vi "pattern.vi"() -> ()   [LabVIEW 2025]
uses:
  ready/Type Def/steps--ring.ctl
panel:
  out "error out":errorcluster
  in  "error in (no error)":errorcluster
  out "VISA resource name out":refnum<visa-resource-name>
  in  "VISA resource name":refnum<visa-resource-name>
  out "ARC value":string
  out "Resulting command":string
  in  "Step":T1=1 min=1 max=99 step=1
  # "Configure ARC Limit"
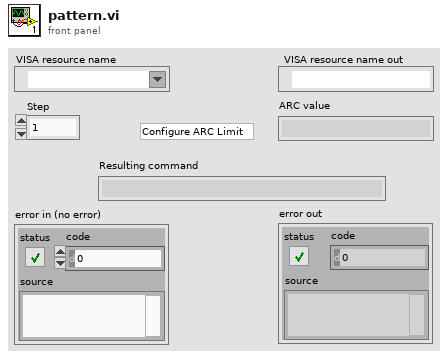
[diagram p1: front panel]
types:
  T1 = typedef "steps--ring.ctl" = u8
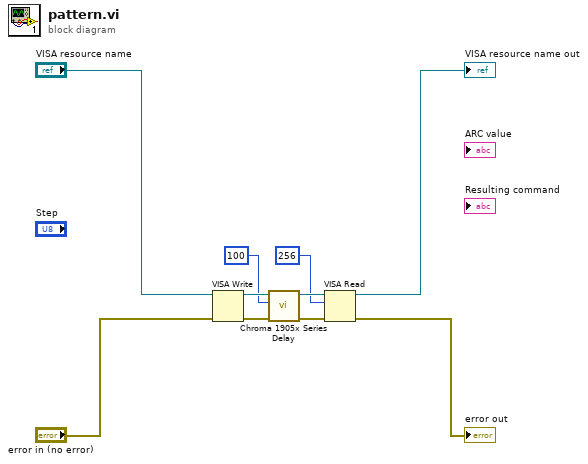
[diagram p0: block diagram]
diagram:
  n1 = VISA Write(VISA resource name="VISA resource name", error in (no error)="error in (no error)") -> (VISA resource name out=w8:refnum<visa-resource-name>, error out=w10:errorcluster)  [unwired: 1 in, 1 out]
  n2 = call "Chroma 1905x Series Delay.vi"("error in (no error)"=w10, "Time Delay [ms]"=u32 100 ("Time Delay ms"), "VISA resource name"=w8) -> ("error out"=w9:errorcluster, "VISA resource name 2"=w7:refnum<visa-resource-name>)  [unwired: 7 in]
  n3 = VISA Read(VISA resource name=w7, byte count=u32 256, error in (no error)=w9) -> (VISA resource name out=→"VISA resource name out":refnum<visa-resource-name>, error out=→"error out":errorcluster)  [unwired: 2 out]
